vi "Read from File.vi"(7 "Channel Direction":string, 8 "error in (no error)":errorcluster, 11 "ConfigFile in":refnum<class "ConfigFile.lvclass">) -> (0 "error out":errorcluster, 2 "Channels":refnum<class "Channel.lvclass">[](array[class]), 3 "ConfigFile out":refnum<class "ConfigFile.lvclass">)   [LabVIEW 2020, in "ImportExport.lvlib" / "ConfigFile.lvclass"]
uses:
  ConfigFile.lvclass
  built/windows/Channel.lvlibp/Channel.lvclass
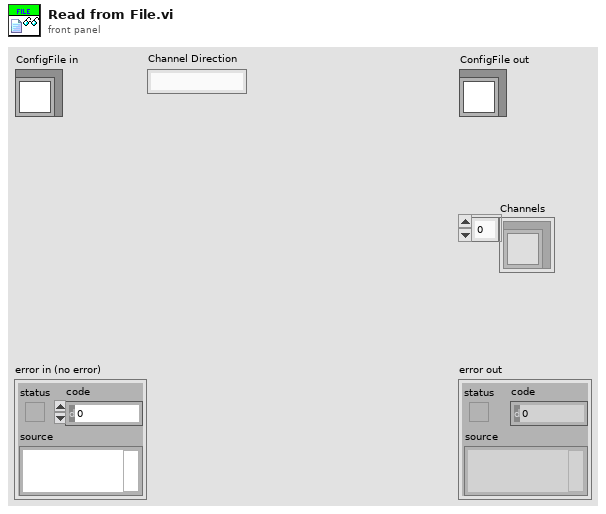
[diagram p1: front panel]
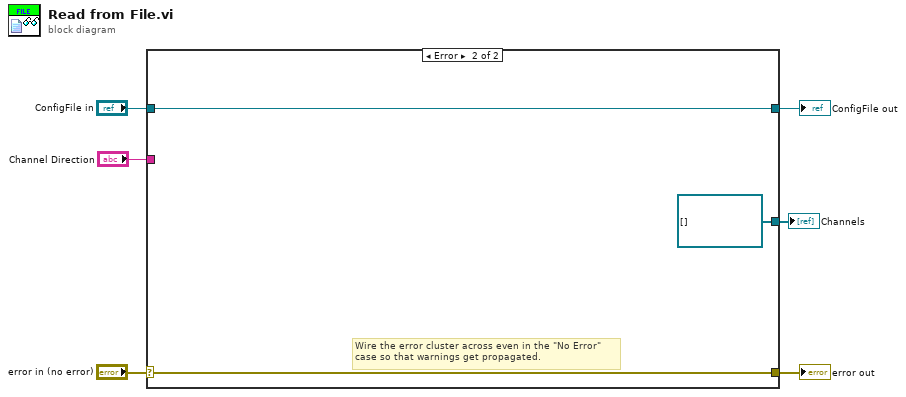
[diagram p0: block diagram]
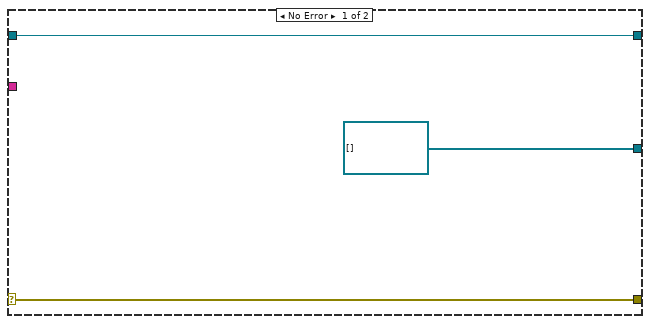
[diagram p2: hidden frame]
diagram:
  n1 = case shown="Error" "error in (no error)" {
    selector: "error in (no error)" -> [w8 w11]
    tunnel: [w8 w11] -> w5
    tunnel: [w9 w12] -> w3
    tunnel: "ConfigFile in" -> [w9 w12]
    tunnel: "Channel Direction" -> [_ _]
    tunnel: [refnum<class "Channel.lvclass">[] [] ("Channels") refnum<class "Channel.lvclass">[] [] ("Channels")] -> w1
    frame No Error {
    }
    frame Error {
      # "Wire the error cluster across even in the \"No Error\"\ncase so that warnings get propagated."
    }
  }
  "error out" <- w5
  "ConfigFile out" <- w3
  "Channels" <- w1
